vi "test_DIO.vi"() -> ()   [LabVIEW 2019]
uses:
  <vilib>/ULx/Create Channel.llb/ULx Create Channel (DO-Digital Output).vi
  <vilib>/ULx/Create Channel.llb/ULx Create Channel (DI-Digital Input).vi
  <vilib>/ULx/Write.llb/ULx Write (Digital Bool 1Line 1Point).vi
  <vilib>/ULx/Read.llb/ULx Read (Digital Bool 1Line 1Point).vi
panel:
  out "error open read":errorcluster
  out "error read":errorcluster
  out "data_read":bool
  in  "digital_input_line":refnum<k21>="Dev0/AuxPort/Di4"
  in  "milliseconds to wait":u32=1000
  out "number":u32=1
  out "error open write":errorcluster
  in  "digital_output_line":refnum<k21>="Dev0/AuxPort/Do0"
  out "error write":errorcluster
  out "data_write":bool
  in  "Stop Button":bool
  # "VI to test the digital input+output of MCC E-TC."
  # "Use DIO0 as the digital output line."
  # "Use DIO4 as the digital input line."
  # "Use pin #28 as GND, if you measure the level of DIO0 or DIO4."
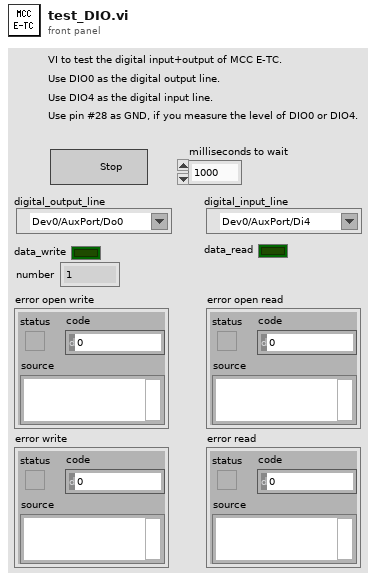
[diagram p1: front panel]
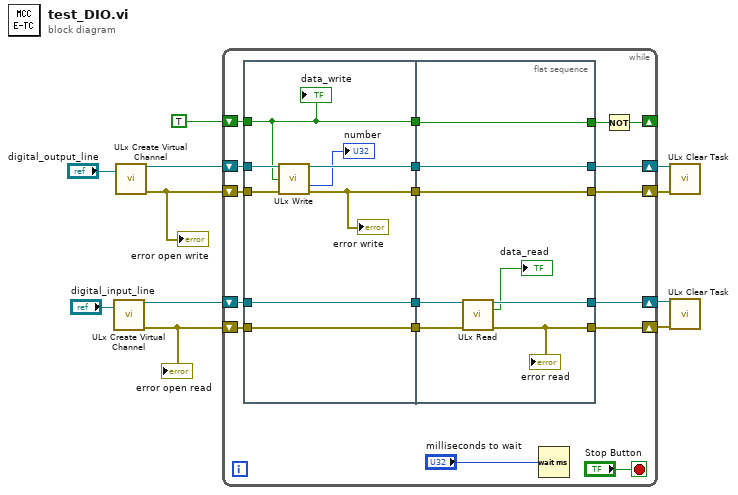
[diagram p0: block diagram]
diagram:
  n1 = call-poly <vilib>:"ULx Create Virtual Channel.vi"("lines"="digital_input_line") -> ("task out"=w4:refnum<k24>, "error out"=w3:errorcluster)  [unwired: 13 in]
  "error open read" <- w3
  n2 = call-poly <vilib>:"ULx Create Virtual Channel.vi"("lines"="digital_output_line") -> ("task out"=w8:refnum<k24>, "error out"=w7:errorcluster)  [unwired: 13 in]
  "error open write" <- w7
  n3 = while {
    shift-right: [w27] -> w9
    shift-left: w8 -> [w28]
    shift-right: [w22] -> w10
    shift-left: w7 -> [w26]
    shift-right: [w25] -> _
    shift-left: TRUE -> [w24]
    shift-right: [w15] -> w2
    shift-left: w4 -> [w17]
    shift-right: [w12] -> w1
    shift-left: w3 -> [w14]
    stop <- "Stop Button" stop-if-true
    n4 = flat-sequence {
      tunnel: w28 -> [w37]
      tunnel: w26 -> [w35]
      tunnel: w24 -> [w32]
      tunnel: [w36] -> w21
      tunnel: [w34] -> w20
      tunnel: [w32] -> w18
      tunnel: w17 -> [w31]
      tunnel: [w31] -> w16
      tunnel: w14 -> [w30]
      tunnel: [w30] -> w13
      tunnel: [w44] -> w22
      tunnel: [w45] -> w27
      tunnel: w21 -> [w45]
      tunnel: w20 -> [w44]
      tunnel: [w43] -> w19
      tunnel: w18 -> [w43]
      tunnel: w16 -> [w42]
      tunnel: [w41] -> w15
      tunnel: w13 -> [w39]
      tunnel: [w38] -> w12
      frame #0 {
        n5 = call-poly <vilib>:"ULx Write.vi"("task in"=w37, "data"=w32, "error in"=w35) -> ("task out"=w36:refnum<k24>, "number of samples written per channel"=→"number":u32, "error out"=w34:errorcluster)  [unwired: 10 in]
        "error write" <- w34
        "data_write" <- w32
      }
      frame #1 {
        n6 = call-poly <vilib>:"ULx Read.vi"("task in"=w42, "error in"=w39) -> ("task out"=w41:refnum<k24>, "data"=→"data_read":bool, "error out"=w38:errorcluster)  [unwired: 11 in]
        "error read" <- w38
      }
    }
    n7 = Wait (ms)(milliseconds to wait="milliseconds to wait") -> ()  [unwired: 1 out]
    n8 = Not(x=w19) -> (.not. x?=w25:bool)
  }
  n9 = call <vilib>:"ULx Clear Task.vi"("task in"=w9, "error in"=w10) -> ()  [unwired: 13 in, 1 out]
  n10 = call <vilib>:"ULx Clear Task.vi"("task in"=w2, "error in"=w1) -> ()  [unwired: 13 in, 1 out]
